vi "Controller.vi"(7 "Controller Values":T1 {"Offset" min=-10.0 max=10.0 step=0.001953125; "Kt" min=0.0 max=0.0; "Ka" min=0.0 max=0.0}, 8 "Error In":errorcluster, 9 "Set Point":dbl, 10 "Position FB":dbl, 11 "Tacho FB":dbl) -> (0 "Error Out":errorcluster, 2 "Controller Out":dbl)   [LabVIEW 2016]
uses:
  Controller Values.ctl
  <vilib>/imath/engines/lvmath2/RunTimeEngine/Managers/WorkSpace/UID Generator.vi
  <vilib>/imath/engines/lvmath2/RunTimeEngine/RunTimeType/NIMS_RunTimeType_From StrictType (excl LVString).vi
  <instcachedir>/0/NIMS_RunTimeType_From StrictType (excl LVString)_BBF44FB49F834B71AF7A14CCEDF8BECD.lvgen/NIMS_RunTimeType_From StrictType (excl LVString)_BBF44FB49F834B71AF7A14CCEDF8BECD_031.vi
  <vilib>/imath/engines/lvmath2/RunTimeEngine/LocalVariableDefStatement/MC_LocalVariableDefStatement_Display.vi
  <vilib>/imath/engines/lvmath2/RunTimeEngine/Managers/SymbolTable/Clear UID.vi
  <vilib>/imath/engines/lvmath2/RunTimeEngine/NodeEndStatement/NIMS_NodeEndStatement_Output.vi
  <instcachedir>/0/NIMS_NodeEndStatement_Output_53EC0D466D134D7ABD903AC30B43404B.lvgen/NIMS_NodeEndStatement_Output_53EC0D466D134D7ABD903AC30B43404B_001.vi
  <vilib>/imath/engines/lvmath2/RunTimeEngine/ErrorHandling/NIMS_Finalize Error.vi
  <vilib>/imath/engines/lvmath2/RunTimeEngine/Managers/SymbolTable/NIMS_WorkSpace.lvlib
panel:
  in  "Max Limit":dbl=10.0
  in  "Min Limit":dbl=-10.0
  out "Limit?":bool=TRUE
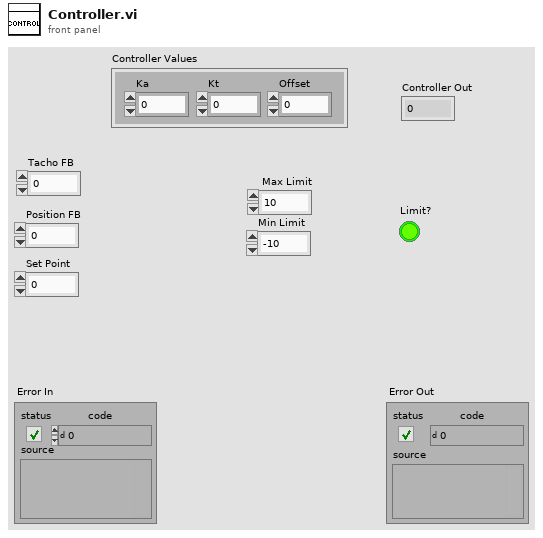
[diagram p1: front panel]
types:
  T1 = typedef "Controller Values.ctl" = cluster{"Ka":dbl, "Kt":dbl, "Offset":dbl}
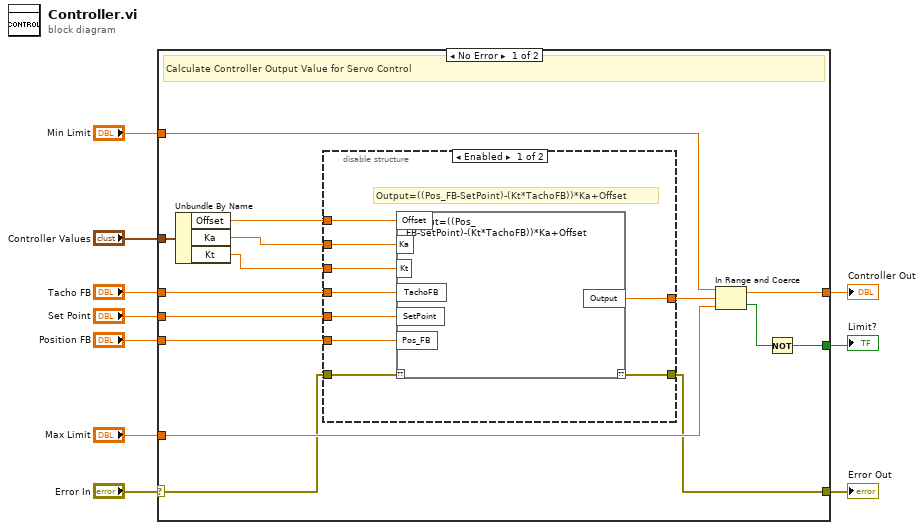
[diagram p0: block diagram]
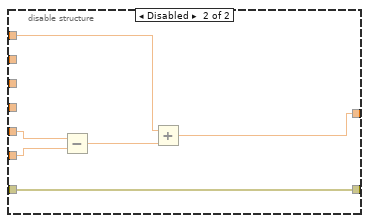
[diagram p2: hidden frame]
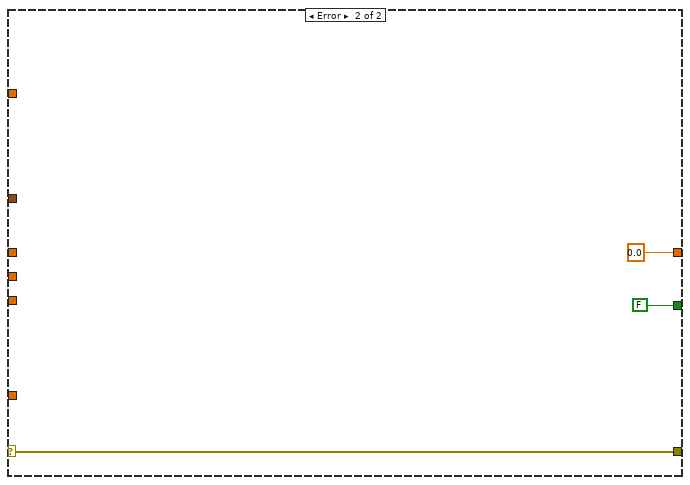
[diagram p3: hidden frame]
diagram:
  n1 = case shown="No Error" "Error In" {
    selector: "Error In" -> [w12 w97]
    tunnel: "Tacho FB" -> [w13 _]
    tunnel: "Controller Values" -> [w23 _]
    tunnel: "Set Point" -> [w24 _]
    tunnel: "Position FB" -> [w25 _]
    tunnel: [w17 0.0 ("Upper Limit (10)")] -> w6
    tunnel: [w11 w97] -> w4
    tunnel: [w20 FALSE] -> w2
    tunnel: "Max Limit" -> [w19 _]
    tunnel: "Min Limit" -> [w14 _]
    frame No Error {
      # "Calculate Controller Output Value for Servo Control"
      n2 = Unbundle By Name(w23) -> ("Offset"=w21:dbl, "Ka"=w22:dbl, "Kt"=w15:dbl)
      n3 = disable-structure shown="Enabled" {
        disable-tunnel: w25 -> [w34 w93]
        disable-tunnel: w24 -> [w33 w94]
        disable-tunnel: w22 -> [w32 _]
        disable-tunnel: w21 -> [w31 w91]
        disable-tunnel: [w30 w90] -> w18
        disable-tunnel: w15 -> [w29 _]
        disable-tunnel: w13 -> [w28 _]
        disable-tunnel: w12 -> [w27 w89]
        disable-tunnel: [w26 w89] -> w11
        frame Enabled {
          # "Output=((Pos_FB-SetPoint)-(Kt*TachoFB))*Ka+Offset"
          n4 = mathscript code="Output=((Pos_FB-SetPoint)-(Kt*TachoFB))*Ka+Offset"("??"=w27, "TachoFB"=w28, "SetPoint"=w33, "Pos_FB"=w34, "Ka"=w32, "Kt"=w29, "Offset"=w31) -> ("??"=w26:errorcluster, "Output"=w30:dbl)
        }
        frame Disabled {
          n5 = Subtract(x=w94, y=w93) -> (x-y=w92:dbl)
          n6 = Add(x=w91, y=w92) -> (x+y=w90:dbl)
        }
      }
      n7 = In Range and Coerce(upper limit=w14, x=w18, lower limit=w19) -> (coerced(x)=w17:dbl, In Range?=w16:bool)
      n8 = Not(x=w16) -> (.not. x?=w20:bool)
    }
    frame Error {
    }
  }
  "Controller Out" <- w6
  "Error Out" <- w4
  "Limit?" <- w2
